vi "Reshape Image (SubVI).vi"(0 "Pixel Data In":u8, 5 "Pixel In Valid?":bool=TRUE, 10 "Block Size":u16=8, 12 "Image Width":u16=512) -> (14 "Pixel Data Out":u8, 19 "Pixel Out Valid?":bool)   [LabVIEW 2014]
uses:
  Controls (FPGA)/Image Block Readout.ctl
  Controls (FPGA)/Image Block Write.ctl
  <vilib>/rvi/Emulation/niFpgaSctlEmulationGetInTimedLoop.vi
  <vilib>/Utility/error.llb/Clear Errors.vi
  <vilib>/rvi/DataTransferAndStorage/Container/Common/niFpgaContainerGetUniqueNameForEmu.vi
  <vilib>/rvi/DataTransferAndStorage/Container/Common/niFpgaContainerSetEmuInfo.vi
  <vilib>/rvi/eio/common/nirviEmuReportErrorAndStop.vi
  <vilib>/rvi/Memory/Memory_Emulation/nirvimemoryFastEmulation.vi
  <vilib>/rvi/Memory/Memory_Emulation/nirvimemoryEmulation.vi
  <vilib>/rvi/Emulation/niFpgaEmulationIsFPGAContextNoSignature.vi
  <vilib>/rvi/Emulation/niFpgaProcessEmulError.vi
  <vilib>/rvi/errors/nirviReportUnexpectedCaseInternalError (U32).vi
  <vilib>/rvi/errors/niFpgaSetErrorForExecOnDevCompSimple.vi
  <vilib>/rvi/FIFO/Fifo_Resource/nirvififoEmulationSetSize.vi
  <vilib>/rvi/FIFO/Fifo_Resource/nirviFifoEmulationQueueMgr.vi
  <instcachedir>/0/nirviFifoEmulationQueueMgr_E5CAEC123FF24DC58D834DCA3CDAA9B5.lvgen/nirviFifoEmulationQueueMgr_E5CAEC123FF24DC58D834DCA3CDAA9B5_002.vi
  <vilib>/rvi/FIFO/Fifo_Resource/nirvififoEmulationDetermineInputValidOut.vi
  <vilib>/rvi/FIFO/Fifo_Resource/nirvififoEmulationCreateLock.vi
  <vilib>/rvi/FIFO/Fifo_Resource/nirvififoEmulationObtainLock.vi
  <vilib>/rvi/FIFO/Fifo_Resource/nirvififoEmulationReleaseLock.vi
  <vilib>/rvi/occurrence/nirviWaitOnOccurrenceBase.vi
  <vilib>/rvi/errors/nirviReportUnexpectedCaseInternalError.vi
  <vilib>/rvi/LocalResourceManager/LocalResourceManager.xnode
  <vilib>/rvi/DataTransferAndStorage/Container/XNode/niFpgaContainer.xnode
  <vilib>/rvi/FIFO/Fifo_Resource/nirvififoEmulationWrite.vi
  <vilib>/rvi/FIFO/Fifo_Resource/nirvififoEmulationRead.vi
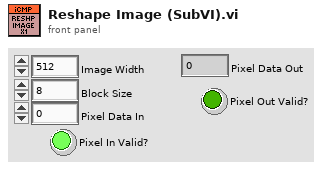
[diagram p1: front panel]
types:
  T1 = typedef "Image Block Readout.ctl" = enum16{"Sync Read", "Read Block Set 1", "Read Block Set 2"}
  T2 = typedef "Image Block Write.ctl" = enum16{"Block 1", "Block 2"}
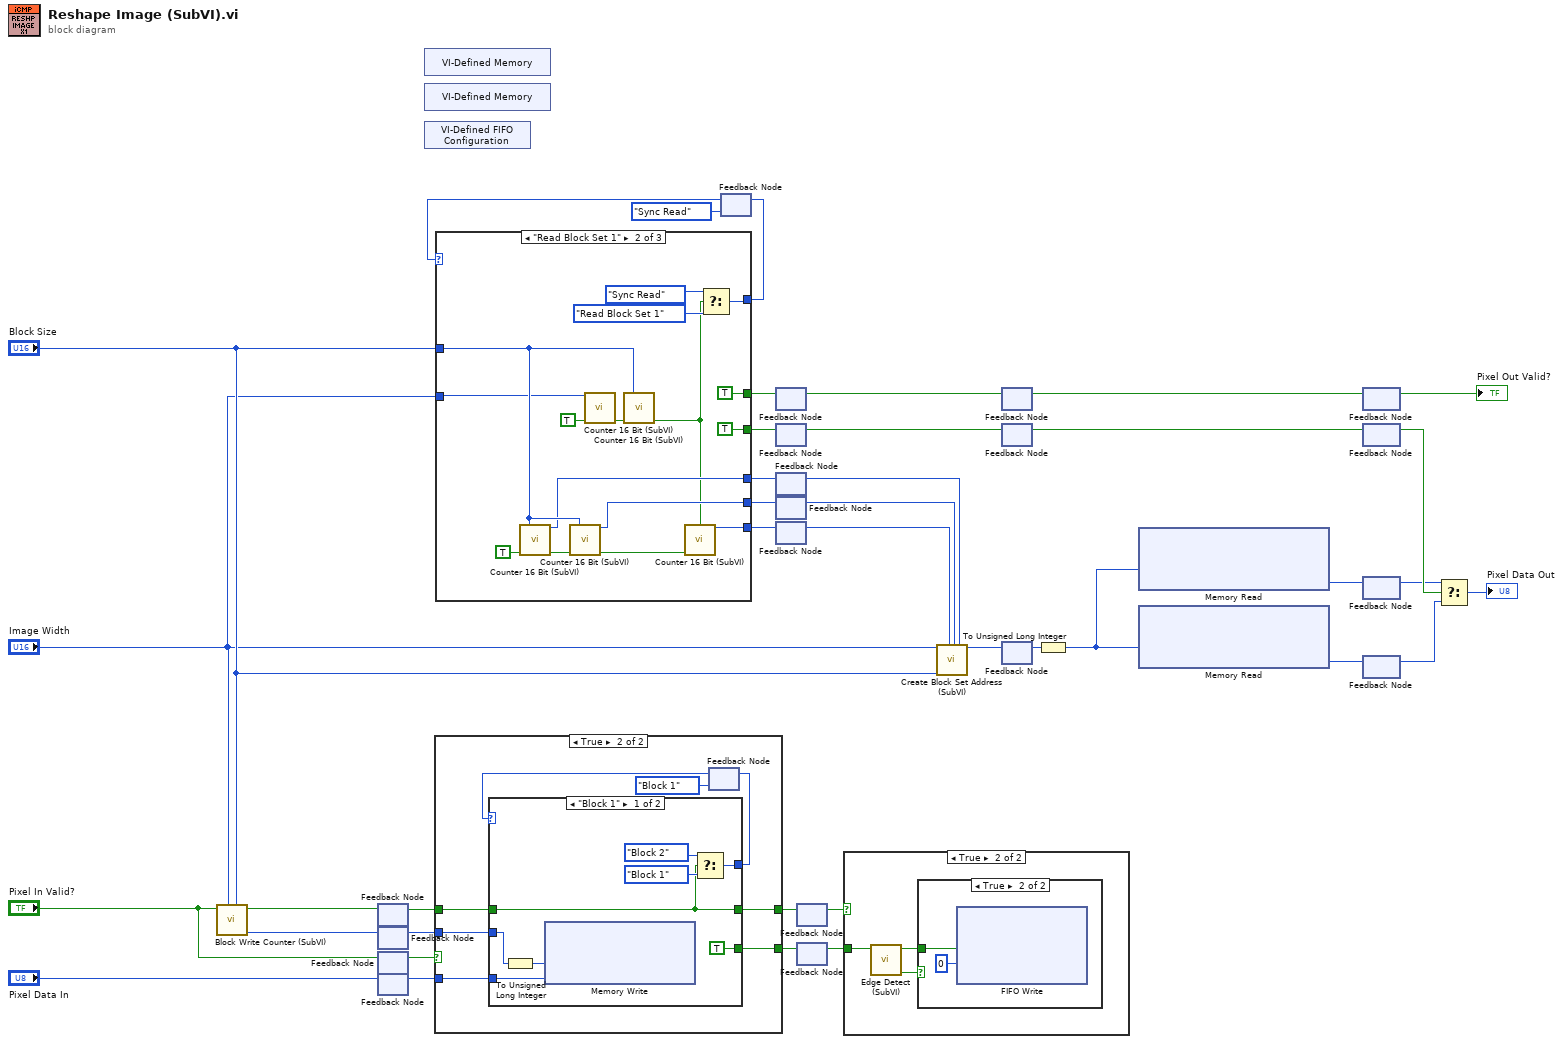
[diagram p0: block diagram]
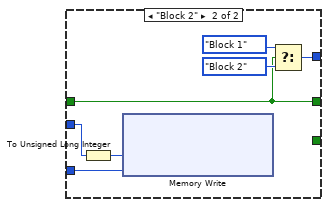
[diagram p5: hidden frame]
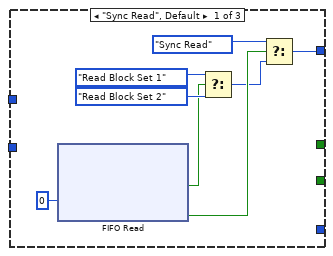
[diagram p6: hidden frame]
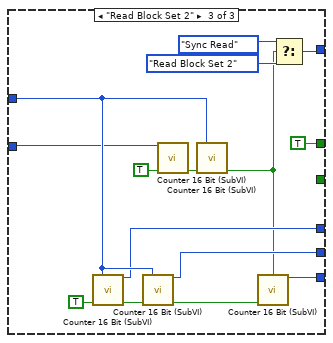
[diagram p7: hidden frame]
diagram:
  n1 = call "Block Write Counter (SubVI).vi"("Block Size"="Block Size", "Image Width"="Image Width", "Pixel Valid?"="Pixel In Valid?") -> ("Count"=w11:u16, "Count End?"=w13:bool)  [unwired: 7 in]
  n2 = feedback-in #1(w13) -> ()
  n3 = feedback #1() -> (w9:bool)  [unwired: 1 in]
  n4 = feedback-in #2(w11) -> ()
  n5 = feedback #2() -> (w8:u16)  [unwired: 1 in]
  n6 = feedback-in #3("Pixel In Valid?") -> ()
  n7 = feedback #3() -> (w7:bool)  [unwired: 1 in]
  n8 = feedback-in #4("Pixel Data In") -> ()
  n9 = feedback #4() -> (w6:u8)  [unwired: 1 in]
  n10 = xnode "VI-Defined Memory"() -> ()  [unwired: 1 out]
  n11 = xnode "VI-Defined Memory"() -> ()  [unwired: 1 out]
  n12 = xnode "VI-Defined FIFO Configuration"() -> ()  [unwired: 1 out]
  n13 = case shown="True" w7 {
    tunnel: w6 -> [_ w44]
    tunnel: w9 -> [_ w43]
    tunnel: w8 -> [_ w42]
    tunnel: [_ w41] -> w5
    tunnel: [_ w40] -> w4
    frame False {
    }
    frame True {
      n14 = feedback #5(Image_Block_Write."Block 1") -> (w46:T2)
      n15 = case shown="\"Block 1\"" w46 {
        tunnel: w42 -> [w55 w62]
        tunnel: w44 -> [w54 w61]
        tunnel: [w50 w57] -> w47
        tunnel: w43 -> [w48 w56]
        tunnel: [w48 w56] -> w41
        tunnel: [TRUE ("Enable") _] -> w40
        frame "Block 1" {
          n16 = To Unsigned Long Integer(number=w55) -> (unsigned 32bit integer=w53:u32)
          n17 = xnode "Memory Write"("Address"=w53, "Data"=w54) -> ()  [unwired: 1 in, 1 out]
          n18 = Select(t=Image_Block_Write."Block 2", s=w48, f=Image_Block_Write."Block 1") -> (s? t:f=w50:T2)
        }
        frame "Block 2" {
          n19 = To Unsigned Long Integer(number=w62) -> (unsigned 32bit integer=w60:u32)
          n20 = xnode "Memory Write"("Address"=w60, "Data"=w61) -> ()  [unwired: 1 in, 1 out]
          n21 = Select(t=Image_Block_Write."Block 1", s=w56, f=Image_Block_Write."Block 2") -> (s? t:f=w57:T2)
        }
      }
      n22 = feedback-in #5(w47) -> ()
    }
  }
  n23 = feedback #6(Image_Block_Readout."Sync Read") -> (w16:T1)
  n24 = case shown="\"Read Block Set 1\"" w16 {
    tunnel: [w69 w83 w98] -> w15
    tunnel: "Block Size" -> [_ w79 w94]
    tunnel: [_ w77 w92] -> w20
    tunnel: [_ w76 w91] -> w21
    tunnel: [_ w75 w90] -> w22
    tunnel: [_ TRUE ("Auto RESET") _] -> w19
    tunnel: [_ TRUE ("Auto RESET") TRUE ("Auto RESET")] -> w18
    tunnel: "Image Width" -> [_ w71 w87]
    frame "Sync Read", Default {
      n25 = xnode "FIFO Read"("Timeout"=0) -> ("Element"=w64:bool, "Timed Out?"=w67:bool)  [unwired: 1 in, 1 out]
      n26 = Select(t=Image_Block_Readout."Read Block Set 1", s=w64, f=Image_Block_Readout."Read Block Set 2") -> (s? t:f=w63:T1)
      n27 = Select(t=Image_Block_Readout."Sync Read", s=w67, f=w63) -> (s? t:f=w69:T1)
    }
    frame "Read Block Set 1" {
      n28 = call "Counter 16 Bit (SubVI).vi"("Max. Count"=w79, "Enable"=TRUE) -> ("Count"=w77:u16, "Count End?"=w81:bool)  [unwired: 11 in, 1 out]
      n29 = call "Counter 16 Bit (SubVI).vi"("Max. Count"=w79, "Enable"=w81) -> ("Count"=w76:u16, "Count End?"=w80:bool)  [unwired: 11 in, 1 out]
      n30 = call "Counter 16 Bit (SubVI).vi"("Max. Count"=w71, "Enable"=TRUE) -> ("Count End?"=w78:bool)  [unwired: 11 in, 2 out]
      n31 = call "Counter 16 Bit (SubVI).vi"("Max. Count"=w79, "Enable"=w78) -> ("Count End?"=w72:bool)  [unwired: 11 in, 2 out]
      n32 = call "Counter 16 Bit (SubVI).vi"("RESET"=w72, "Enable"=w80) -> ("Count"=w75:u16)  [unwired: 11 in, 2 out]
      n33 = Select(t=Image_Block_Readout."Sync Read", s=w72, f=Image_Block_Readout."Read Block Set 1") -> (s? t:f=w83:T1)
    }
    frame "Read Block Set 2" {
      n34 = call "Counter 16 Bit (SubVI).vi"("Max. Count"=w94, "Enable"=TRUE) -> ("Count"=w92:u16, "Count End?"=w96:bool)  [unwired: 11 in, 1 out]
      n35 = call "Counter 16 Bit (SubVI).vi"("Max. Count"=w94, "Enable"=w96) -> ("Count"=w91:u16, "Count End?"=w95:bool)  [unwired: 11 in, 1 out]
      n36 = call "Counter 16 Bit (SubVI).vi"("Max. Count"=w87, "Enable"=TRUE) -> ("Count End?"=w93:bool)  [unwired: 11 in, 2 out]
      n37 = call "Counter 16 Bit (SubVI).vi"("Max. Count"=w94, "Enable"=w93) -> ("Count End?"=w88:bool)  [unwired: 11 in, 2 out]
      n38 = call "Counter 16 Bit (SubVI).vi"("RESET"=w88, "Enable"=w95) -> ("Count"=w90:u16)  [unwired: 11 in, 2 out]
      n39 = Select(t=Image_Block_Readout."Sync Read", s=w88, f=Image_Block_Readout."Read Block Set 2") -> (s? t:f=w98:T1)
    }
  }
  n40 = feedback-in #6(w15) -> ()
  n41 = feedback #7() -> (w27:bool)  [unwired: 1 in]
  n42 = feedback-in #7(w18) -> ()
  n43 = feedback #8() -> (w28:bool)  [unwired: 1 in]
  n44 = feedback-in #8(w19) -> ()
  n45 = feedback #9() -> (w23:u16)  [unwired: 1 in]
  n46 = feedback-in #9(w20) -> ()
  n47 = feedback #10() -> (w24:u16)  [unwired: 1 in]
  n48 = feedback-in #10(w21) -> ()
  n49 = feedback #11() -> (w25:u16)  [unwired: 1 in]
  n50 = feedback-in #11(w22) -> ()
  n51 = feedback-in #12(w5) -> ()
  n52 = feedback #12() -> (w3:bool)  [unwired: 1 in]
  n53 = feedback-in #13(w4) -> ()
  n54 = feedback #13() -> (w2:bool)  [unwired: 1 in]
  n55 = case shown="True" w3 {
    tunnel: w2 -> [_ w102]
    frame False {
    }
    frame True {
      n56 = call "Edge Detect (SubVI).vi"("TTL In"=w102) -> ("Edge?"=w104:bool, "Rising Edge"=w103:bool)  [unwired: 8 in, 1 out]
      n57 = case shown="True" w104 {
        tunnel: w103 -> [_ w105]
        frame False {
        }
        frame True {
          n58 = xnode "FIFO Write"("Element"=w105, "Timeout"=0) -> ()  [unwired: 1 in, 2 out]
        }
      }
    }
  }
  n59 = call "Create Block Set Address (SubVI).vi"("Image Width"="Image Width", "Block Size"="Block Size", "Block N"=w25, "Block Y"=w24, "Block X"=w23) -> ("Address"=w26:u16)  [unwired: 14 in]
  n60 = feedback #14() -> (w33:bool)  [unwired: 1 in]
  n61 = feedback-in #14(w27) -> ()
  n62 = feedback #15() -> (w34:bool)  [unwired: 1 in]
  n63 = feedback-in #15(w28) -> ()
  n64 = feedback #16() -> (w29:u16)  [unwired: 1 in]
  n65 = feedback-in #16(w26) -> ()
  n66 = To Unsigned Long Integer(number=w29) -> (unsigned 32bit integer=w30:u32)
  n67 = xnode "Memory Read"("Address"=w30) -> ("Data"=w32:u8)  [unwired: 1 in, 1 out]
  n68 = xnode "Memory Read"("Address"=w30) -> ("Data"=w31:u8)  [unwired: 1 in, 1 out]
  n69 = feedback #17() -> (→"Pixel Out Valid?":bool)  [unwired: 1 in]
  n70 = feedback-in #17(w33) -> ()
  n71 = feedback #18() -> (w38:bool)  [unwired: 1 in]
  n72 = feedback-in #18(w34) -> ()
  n73 = feedback #19() -> (w36:u8)  [unwired: 1 in]
  n74 = feedback-in #19(w32) -> ()
  n75 = feedback #20() -> (w37:u8)  [unwired: 1 in]
  n76 = feedback-in #20(w31) -> ()
  n77 = Select(t=w36, s=w38, f=w37) -> (s? t:f=→"Pixel Data Out":u8)
